vi "Channel ID to Tree Items.vi"(8 "error in (no error)":errorcluster, 9 "Channel ID":string, 11 "Application Data in":T2) -> (0 "error out":errorcluster, 1 "Settings":T1, 2 "Item":T1, 3 "Application Data out":T2)   [LabVIEW 2017, in "DSF Simple Explorer.lvlib"]
uses:
  DSF Configuration.llb/DSF Simple Explorer.lvlib
  Application Data.ctl
  Windows/DSF Core.lvlibp/Classes/Configuration/Configuration Session.lvclass
  View Mode.ctl
  Tree Item.ctl
  Tree Item Type.ctl
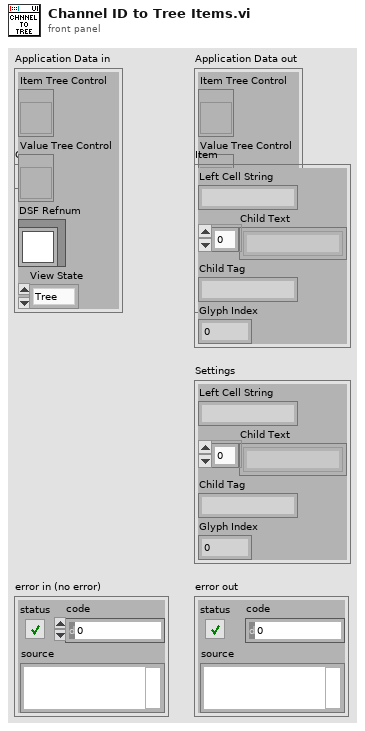
[diagram p1: front panel]
types:
  T1 = typedef "DSF Simple Explorer.lvlib/Tree Item.ctl" = cluster{"Left Cell String":string, "Child Text":string[], "Child Tag":string, "Glyph Index":i32}
  T2 = typedef "DSF Simple Explorer.lvlib/Application Data.ctl" = cluster{"Item Tree Control":refnum<vi>, "Value Tree Control":refnum<vi>, "DSF Refnum":refnum<class "Configuration Session.lvclass">, "View State":T3}
  T3 = typedef "DSF Simple Explorer.lvlib/View Mode.ctl" = enum16{"Tree", "List"}
  T4 = typedef "DSF Simple Explorer.lvlib/Tree Item Type.ctl" = enum16{"Plugin", "Group", "Transfer", "Channel", "Setting"}
  T5 = typedef "DSF Core.lvlibp/DSF Channel Info.ctl" = cluster{"string buffer offset":u64, "string data type":T6, "engine data type":T6, "settings id":string, "units":string}
  T6 = typedef "DSF Core.lvlibp/DSF Data Type.ctl" = enum8{"Bool", "SGL", "DBL", "I8", "I16", "I32", "I64", "U8", "U16", "U32", "U64"}
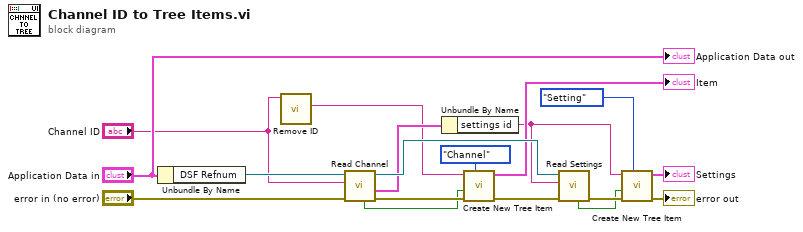
[diagram p0: block diagram]
diagram:
  n1 = Unbundle By Name("Application Data in") -> ("DSF Refnum"=w9:refnum<class "Configuration Session.lvclass">)
  n2 = call "Remove ID.vi"("id string"="Channel ID") -> ("name"=w2:string)  [unwired: 8 in, 2 out]
  n3 = call "Read Channel.vi"("error in (no error)"="error in (no error)", "Channel ID"="Channel ID", "Configuration Session in"=w9) -> ("error out"=w13:errorcluster, "value"=w10:T5, "Configuration Session out"=w11:refnum<class "Configuration Session.lvclass">, "found?"=w6:bool)  [unwired: 5 in]
  n4 = Unbundle By Name(w10) -> ("settings id"=w5:string)
  n5 = call "Create New Tree Item.vi"("Item Type"=Tree_Item_Type."Channel", "error in"=w13, "found?"=w6, "Left Cell String"=w2) -> ("error out"=w14:errorcluster, "Item"=→"Item":T1)  [unwired: 6 in]
  n6 = call "Read Settings.vi"("error in (no error)"=w14, "Settings ID"=w5, "Configuration Session in"=w11) -> ("error out"=w15:errorcluster, "found?"=w4:bool)  [unwired: 5 in, 2 out]
  n7 = call "Create New Tree Item.vi"("Item Type"=Tree_Item_Type."Setting", "error in"=w15, "found?"=w4, "Left Cell String"=w5) -> ("error out"=→"error out":errorcluster, "Item"=→"Settings":T1)  [unwired: 6 in]
  "Application Data out" <- "Application Data in"
